vi "Pre Launch Init.vi"(11 "CS++SVMonitor in":refnum<class "CS++SVMonitor.lvclass">) -> (0 "error out":errorcluster, 3 "CS++SVMonitor out":refnum<class "CS++SVMonitor.lvclass">)   [LabVIEW 2014, in "CS++SVMonitor.lvlib" / "CS++SVMonitor.lvclass"]
doc: "(<B>Filename</B>: Actor Framework.lvlib:Actor.lvclass:Pre Launch Init.vi)\n\nDefines behavior that occurs after the Launch Actor method is invoked but before the actor's Actor Core method begins running.\n\nThe Pre Launch Init method is guaranteed to finish before the Launch Actor method returns to its caller and before the actor itself receives any messages. Any references that the Pre Launch Init method obtains are guaranteed to have the same lifetime as the actor itself. Any errors that the Pre Launch Init method returns will abort the launch.\n\nBy default, this method does nothing. A descendant class may override it to define behavior."
uses:
  CS++SVMonitor.lvclass
  <vilib>/ActorFramework/Message Enqueuer/Message Enqueuer.lvclass
  CS++PVMonitor Messages/CS++PVUpdate Msg/CS++PVUpdate Msg.lvclass
  CS++SVMonitor.lvclass/CS++SVMonitor.ctl
  CS++PVMonitor/CS++PVMonitor.lvclass
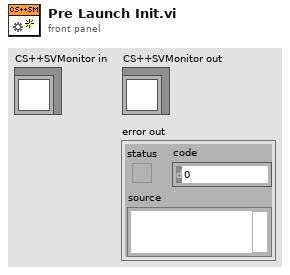
[diagram p1: front panel]
types:
  T1 = cluster{"SV Refnums":refnum<k21>[], "PV Connections":cluster{"PV URL":string, "Observers":cluster{"Enqueuer":refnum<class "Message Enqueuer.lvclass">, "CS++PVUpdate Msg":refnum<class "CS++PVUpdate Msg.lvclass">}[]}[]}
  T2 = cluster{"Stop":refnum<user-event>, "PV Connections":refnum<user-event>}
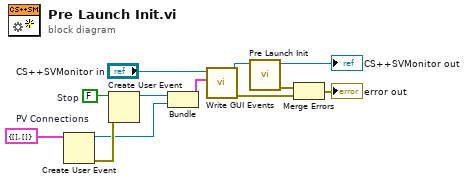
[diagram p0: block diagram]
diagram:
  w8 = T1 {"SV Refnums"=[], "PV Connections"=[]}  # PV Connections
  w10 = FALSE  # Stop
  n1 = Create User Event(user event datatype=w8) -> (user event=w6:refnum<user-event>, error out=w9:errorcluster)  [unwired: 1 in]
  n2 = Create User Event(user event datatype=w10, error in=w9) -> (user event=w7:refnum<user-event>)  [unwired: 1 out]
  n3 = Bundle("Stop"=w7, "PV Connections"=w6) -> (w3:T2)  [unwired: 1 in]
  n4 = call "Write GUI Events.vi"("GUI Events"=w3, "CS++SVMonitor in"="CS++SVMonitor in") -> ("error out"=w1:errorcluster, "CS++SVMonitor out"=w4:refnum<class "CS++SVMonitor.lvclass">)  [unwired: 8 in]
  n5 = call-parent "Pre Launch Init.vi"("CS++BaseActor in"=w4) -> ("error out"=w12:errorcluster, "CS++BaseActor out"=→"CS++SVMonitor out":refnum<class "CS++SVMonitor.lvclass">)  [unwired: 9 in]
  n6 = Merge Errors(w12, w1) -> (→"error out":errorcluster)
